vi "Add Test Suite XML Tag.vi"(8 "error in (no error)":errorcluster, 10 "Suite Name":string, 11 "Reports.lvlib:XML Report.lvclass":refnum<class "XML Report.lvclass">) -> (0 "error out":errorcluster, 3 "output cluster":refnum<class "XML Report.lvclass">)   [LabVIEW 2020, in "Reports.lvlib" / "XML Report.lvclass"]
doc: "Add a new element to an existing DOM document."
uses:
  XML Report.lvclass
  XML Report.lvclass/XML Report.ctl
  <resource>/objmgr/DOMUserDefRef.rc
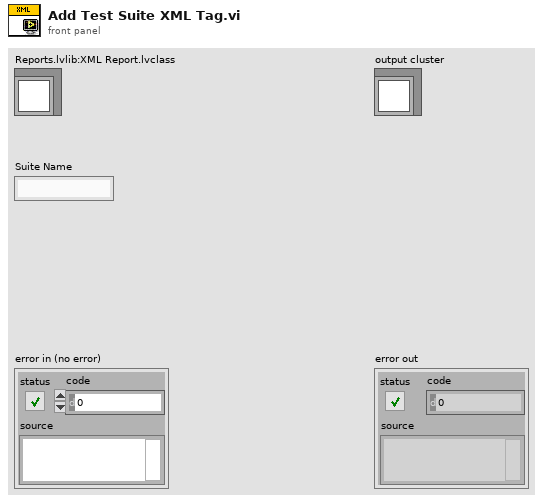
[diagram p1: front panel]
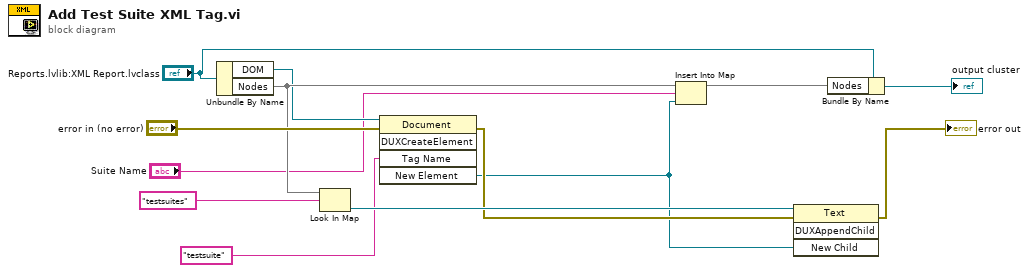
[diagram p0: block diagram]
diagram:
  n1 = Unbundle By Name("Reports.lvlib:XML Report.lvclass") -> ("DOM"=w5:refnum<k20>, "Nodes"=w10:map{string, refnum<k20>})
  n2 = Look In Map(map=w10, key="testsuites" ("Suite Name")) -> (value=w11:refnum<k20>)  [unwired: 1 in, 1 out]
  n3 = invoke class="Document" method="DUXCreateElement"(reference=w5, error in="error in (no error)", "Tag Name"="testsuite") -> (error out=w6:errorcluster, "New Element"=w4:refnum<k20>)  [unwired: 2 in, 3 out]
  n4 = Insert Into Map(map in=w10, key="Suite Name", value=w4) -> (map out=w8:map{string, refnum<k20>})  [unwired: 2 out]
  n5 = invoke class="Text" method="DUXAppendChild"(reference=w11, error in=w6, "New Child"=w4) -> (error out=→"error out":errorcluster)  [unwired: 1 in, 3 out]
  n6 = Bundle By Name(cluster="Reports.lvlib:XML Report.lvclass", "Nodes"=w8) -> (→"output cluster":refnum<class "XML Report.lvclass">)
